vi "Send CMD_M1.vi"(4 "Direction M1":bool, 5 "Speed (mm/s) M1":dbl, 6 "SERVO ON CMD M1":bool, 7 "STM Done Bit":bool, 8 "Home Calling M1":bool, 9 "Mode M1":i32, 10 "Travel (mm)M1":dbl, 11 "Bool Refnum":refnum<vi>) -> ()   [LabVIEW 2015]
uses:
  Project Setup/Globle Variable/GR_Servo.vi
  Galobal variable_TI.vi
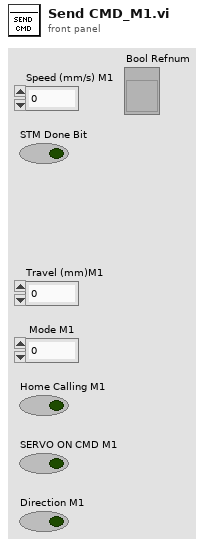
[diagram p1: front panel]
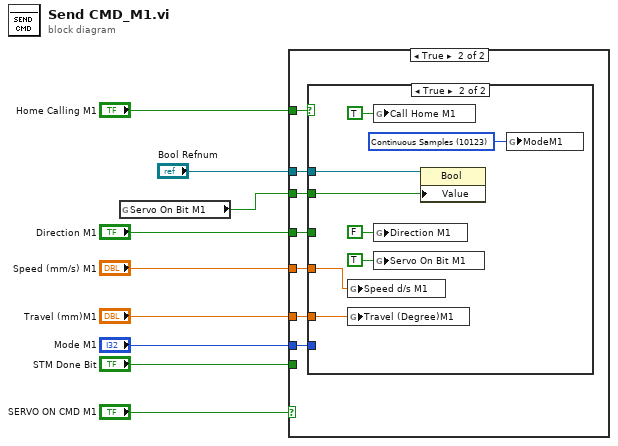
[diagram p0: block diagram]
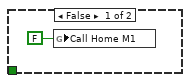
[diagram p2: hidden frame]
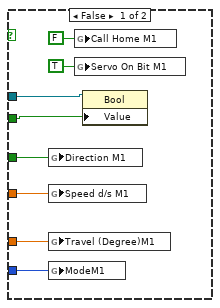
[diagram p3: hidden frame]
diagram:
  n1 = global read "GR_Servo.vi" "Servo On Bit M1"() -> (w1:bool)
  n2 = case shown="True" "SERVO ON CMD M1" {
    tunnel: "STM Done Bit" -> [_ _]
    tunnel: "Mode M1" -> [_ w17]
    tunnel: "Direction M1" -> [_ w16]
    tunnel: "Speed (mm/s) M1" -> [_ w15]
    tunnel: "Travel (mm)M1" -> [_ w14]
    tunnel: "Home Calling M1" -> [_ w13]
    tunnel: "Bool Refnum" -> [_ w12]
    tunnel: w1 -> [_ w11]
    frame False {
      n3 = global write "Galobal variable_TI.vi" "Call Home M1"(FALSE ("Call Home M1")) -> ()
    }
    frame True {
      n4 = case shown="True" w13 {
        tunnel: w17 -> [w24 _]
        tunnel: w16 -> [w21 _]
        tunnel: w15 -> [w23 w30]
        tunnel: w14 -> [w22 w29]
        tunnel: w12 -> [w19 w27]
        tunnel: w11 -> [w18 w26]
        frame False {
          n5 = global write "GR_Servo.vi" "Direction M1"(w21) -> ()
          n6 = global write "GR_Servo.vi" "Speed d/s M1"(w23) -> ()
          n7 = global write "GR_Servo.vi" "Travel (Degree)M1"(w22) -> ()
          n8 = global write "GR_Servo.vi" "ModeM1"(w24) -> ()
          n9 = global write "Galobal variable_TI.vi" "Call Home M1"(FALSE ("Call Home M1")) -> ()
          n10 = global write "GR_Servo.vi" "Servo On Bit M1"(TRUE ("Servo On Bit")) -> ()
          n11 = property class="Bool"(reference=w19, "Value"=w18) -> ()  [unwired: 1 in, 2 out]
        }
        frame True {
          w32 = 10123 items=["Finite Samples"=10178, "Continuous Samples"=10123, "Hardware Timed Single Point"=12522] ("ModeM1")
          n12 = global write "GR_Servo.vi" "Speed d/s M1"(w30) -> ()
          n13 = global write "GR_Servo.vi" "Travel (Degree)M1"(w29) -> ()
          n14 = global write "Galobal variable_TI.vi" "Call Home M1"(TRUE ("Call Home M1")) -> ()
          n15 = global write "GR_Servo.vi" "Direction M1"(FALSE ("Direction M1")) -> ()
          n16 = global write "GR_Servo.vi" "Servo On Bit M1"(TRUE ("Servo On Bit")) -> ()
          n17 = property class="Bool"(reference=w27, "Value"=w26) -> ()  [unwired: 1 in, 2 out]
          n18 = global write "GR_Servo.vi" "ModeM1"(w32) -> ()
        }
      }
    }
  }
